vi "SIFS_ReadPostionAndStatus.vi"(0 "VISA resource name":refnum<visa-resource-name>, 2 "ID":string, 3 "FATOR":dbl) -> (1 "Status Word":bool[](array[boolean]), 5 "Position":dbl, 6 "Switch 3":bool, 7 "Switch 2 Homing":bool, 8 "error out":errorcluster, 9 "Switch 1 Home":bool, 10 "Running when TRUE":bool)   [LabVIEW 2012]
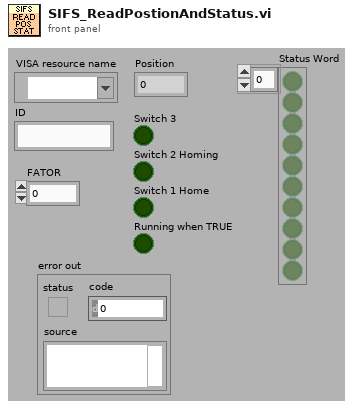
[diagram p1: front panel]
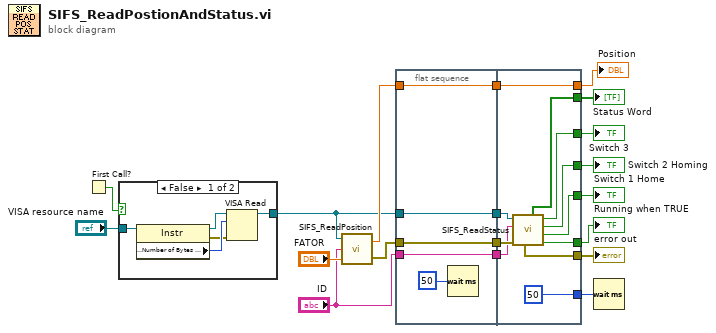
[diagram p0: block diagram]
diagram:
  n1 = First Call?() -> (First Call?: T/F=w8:bool)
  n2 = case shown="False" w8 {
    tunnel: "VISA resource name" -> [w21 w25]
    tunnel: [w20 w25] -> w3
    frame False {
      n3 = property class="Instr"(reference=w21) -> (reference out=w24:refnum<visa-resource-name>, error out=w22:errorcluster, "Serial Settings:Number of Bytes at Serial Port"=w23:u32)  [unwired: 1 in]
      n4 = VISA Read(VISA resource name=w24, byte count=w23, error in (no error)=w22) -> (VISA resource name out=w20:refnum<visa-resource-name>)  [unwired: 3 out]
    }
    frame True {
    }
  }
  n5 = call "SIFS_ReadPosition.vi"("FATOR"="FATOR", "ID"="ID", "VISA resource name"=w3) -> ("error out"=w4:errorcluster, "Position"=w5:dbl)
  n6 = flat-sequence {
    tunnel: [w27] -> w15
    tunnel: [w29] -> w13
    tunnel: [w28] -> w10
    tunnel: w5 -> [w29]
    tunnel: w4 -> [w28]
    tunnel: w3 -> [w27]
    tunnel: "ID" -> [w26]
    tunnel: [w26] -> w1
    tunnel: w15 -> [w41]
    tunnel: [w40] -> w19
    tunnel: [w39] -> w18
    tunnel: [w38] -> w17
    tunnel: [w37] -> w16
    tunnel: [u32 50 ("milliseconds to wait")] -> w14
    tunnel: [w35] -> w12
    tunnel: w13 -> [w35]
    tunnel: [w34] -> w11
    tunnel: w10 -> [w33]
    tunnel: [w32] -> w7
    tunnel: w1 -> [w31]
    frame #0 {
      n7 = Wait (ms)(milliseconds to wait=u32 50) -> ()  [unwired: 1 out]
    }
    frame #1 {
      n8 = call "SIFS_ReadStatus.vi"("error in"=w33, "ID"=w31, "VISA resource name"=w41) -> ("Running when true"=w40:bool, "Switch 1 Home"=w39:bool, "Switch 2 Homing"=w38:bool, "Switch 3"=w37:bool, "Status Word"=w32:bool[], "error out"=w34:errorcluster)  [unwired: 3 out]
    }
  }
  n9 = Wait (ms)(milliseconds to wait=w14) -> ()  [unwired: 1 out]
  "Position" <- w12
  "Switch 2 Homing" <- w17
  "Switch 3" <- w16
  "Switch 1 Home" <- w18
  "Running when TRUE" <- w19
  "error out" <- w11
  "Status Word" <- w7
